vi "verification-login.vi"(6 "Username":refnum<vi>, 9 "Staff-Admin-Tabs":refnum<vi>, 10 "Password":refnum<vi>, 11 "User FP":refnum<vi>) -> (3 "Login Success?":bool)   [LabVIEW 2021]
uses:
  <vilib>/Utility/file.llb/Read Delimited Spreadsheet (string).vi
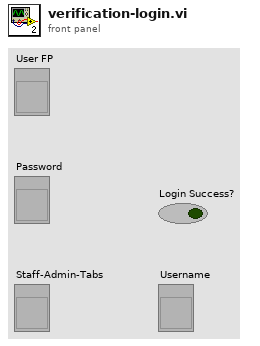
[diagram p1: front panel]
types:
  T1 = enum32{"Controls", "Login", "Home", "Register Admin", "Server Status"}
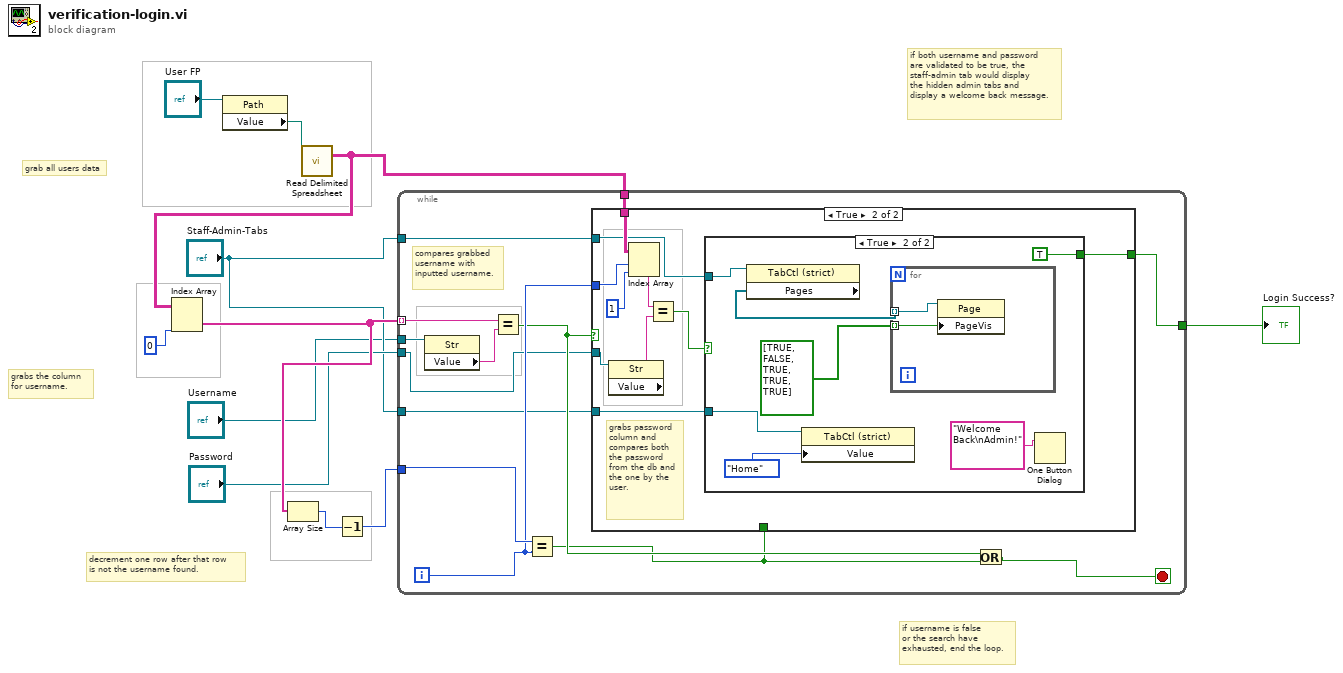
[diagram p0: block diagram]
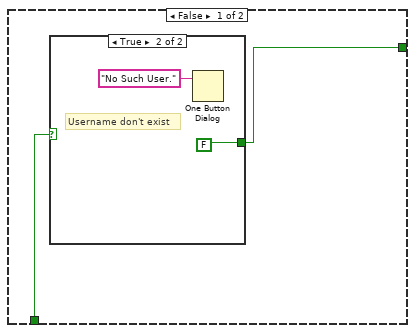
[diagram p2: hidden frame]
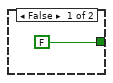
[diagram p3: hidden frame]
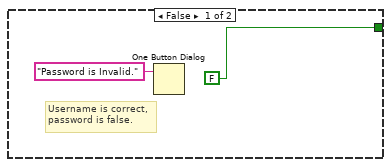
[diagram p4: hidden frame]
diagram:
  # "if username is false\nor the search have\nexhausted, end the loop."
  # "if both username and password\nare validated to be true, the\nstaff-admin tab would display\nthe hidden admin tabs and\ndisplay a welcome back message."
  # "decrement one row after that row\nis not the username found."
  # "grabs the column \nfor username."
  # "grab all users data"
  n1 = property class="Path"(reference="User FP") -> ("Value"=w7:path)  [unwired: 1 in, 2 out]
  n2 = call-poly <vilib>:"Read Delimited Spreadsheet.vi"("file path (dialog if empty)"=w7) -> ("all rows"=w11:string[][])  [unwired: 9 in, 5 out]
  n3 = Index Array(array=w11, index (col)=0 ("disabled index (col)")) -> (element=w9:string[])  [unwired: 1 in]
  n4 = Array Size(array=w9) -> (size(s)=w10:i32)
  n5 = Decrement(x=w10) -> (x-1=w1:i32)
  n6 = while {
    tunnel: w9 -> [w22] mode=indexing
    tunnel: w1 -> [w24]
    tunnel: w11 -> [w17]
    tunnel: "Password" -> [w16]
    tunnel: "Staff-Admin-Tabs" -> [w15]
    tunnel: "Staff-Admin-Tabs" -> [w14]
    tunnel: "Username" -> [w13]
    tunnel: [w12] -> w2
    i -> [w23]
    stop <- w20 stop-if-true
    # "compares grabbed \nusername with \ninputted username."
    n7 = property class="Str"(reference=w13) -> ("Value"=w21:string)  [unwired: 1 in, 2 out]
    n8 = Equal?(x=w22, y=w21) -> (x = y?=w19:bool)
    n9 = Equal?(x=w24, y=w23) -> (x = y?=w18:bool)
    n10 = case shown="True" w19 {
      tunnel: w23 -> [_ w38]
      tunnel: w18 -> [w26 _]
      tunnel: w17 -> [_ w39]
      tunnel: [w25 w33] -> w12
      tunnel: w16 -> [_ w32]
      tunnel: w15 -> [_ w31]
      tunnel: w14 -> [_ w30]
      frame False {
        n11 = case shown="True" w26 {
          tunnel: [FALSE FALSE] -> w25
          frame False {
          }
          frame True {
            # "Username don't exist"
            n12 = One Button Dialog(message="No Such User.") -> ()  [unwired: 1 in, 1 out]
          }
        }
      }
      frame True {
        # "grabs password\ncolumn and\ncompares both\nthe password\nfrom the db and\nthe one by the\nuser."
        n13 = property class="Str"(reference=w32) -> ("Value"=w35:string)  [unwired: 1 in, 2 out]
        n14 = Index Array(array=w39, index (row)=w38, index (col)=1 ("disabled index (col)")) -> (element=w36:string)
        n15 = Equal?(x=w36, y=w35) -> (x = y?=w34:bool)
        n16 = case shown="True" w34 {
          tunnel: [FALSE TRUE] -> w33
          tunnel: w31 -> [_ w43]
          tunnel: w30 -> [_ w42]
          frame False {
            # "Username is correct,\npassword is false."
            n17 = One Button Dialog(message="Password is Invalid.") -> ()  [unwired: 1 in, 1 out]
          }
          frame True {
            n18 = property on="Property Node" class="TabCtl (strict)"(reference=w43) -> ("Pages"=w48:refnum<vi>[])  [unwired: 1 in, 2 out]
            n19 = property on="Property Node" class="TabCtl (strict)"(reference=w42, "Value"=T1."Home" ("Staff-Admin-Tabs")) -> ()  [unwired: 1 in, 2 out]
            n20 = for {
              tunnel: w48 -> [w50] mode=indexing
              tunnel: bool[] [TRUE, FALSE, TRUE, TRUE, TRUE] -> [w49] mode=indexing
              n21 = property class="Page"(reference=w50, "PageVis"=w49) -> ()  [unwired: 1 in, 2 out]
            }
            n22 = One Button Dialog(message="Welcome Back\nAdmin!") -> ()  [unwired: 1 in, 1 out]
          }
        }
      }
    }
    n23 = Or(x=w19, y=w18) -> (x .or. y?=w20:bool)
  }
  "Login Success?" <- w2
